vi "Clear Messages.vi"(8 "error in (no error)":errorcluster, 10 "Data":variant, 11 "CheckPasswordUI in":refnum<class "CheckPasswordUI.lvclass">) -> (0 "error out":errorcluster, 3 "CheckPasswordUI out":refnum<class "CheckPasswordUI.lvclass">)   [LabVIEW 2021, in "CheckPasswordUI.lvclass"]
uses:
  CheckPasswordUI.lvclass
  CheckPasswordUI.lvclass/CheckPasswordUI.ctl
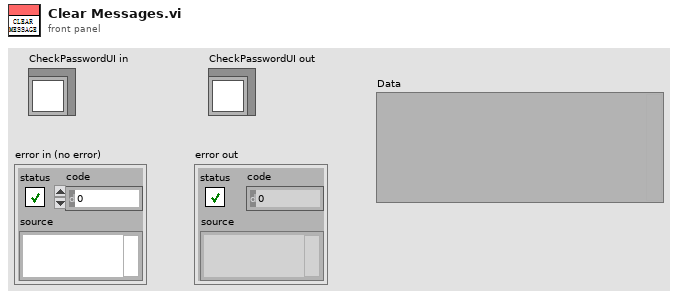
[diagram p1: front panel]
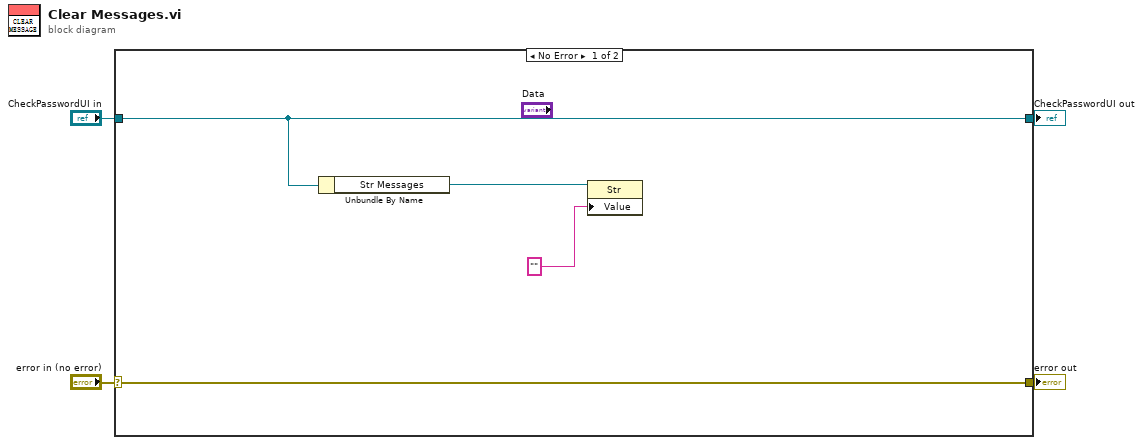
[diagram p0: block diagram]
diagram:
  n1 = case shown="No Error" "error in (no error)" {
    selector: "error in (no error)" -> [w8 w10]
    tunnel: [w8 w10] -> w3
    tunnel: [w5 w9] -> w1
    tunnel: "CheckPasswordUI in" -> [w5 w9]
    frame No Error {
      n2 = Unbundle By Name(w5) -> ("Str Messages"=w6:refnum<vi>)
      n3 = property class="Str"(reference=w6, "Value"="") -> ()  [unwired: 1 in, 2 out]
    }
    frame Error {
    }
  }
  "error out" <- w3
  "CheckPasswordUI out" <- w1
